vi "Init Actor Core.vi"(8 "error in (no error)":errorcluster, 11 "Measure Object in":refnum<class "Instrument Actor.lvclass">) -> (0 "error out":errorcluster, 3 "Measure Object out":refnum<class "Instrument Actor.lvclass">)   [LabVIEW 2021, in "Instrument Actor.lvclass"]
uses:
  Instrument Actor.lvclass
  Instrument Actor.lvclass/Instrument Actor.ctl
  Worker/Worker.lvclass
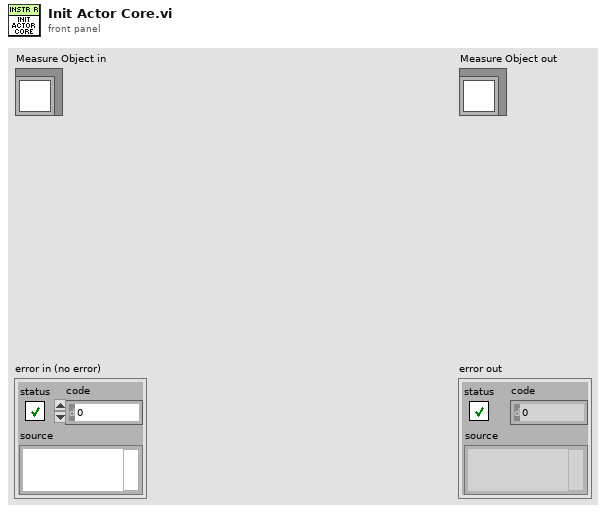
[diagram p1: front panel]
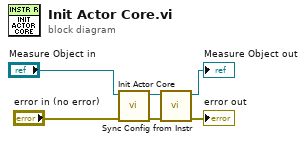
[diagram p0: block diagram]
diagram:
  n1 = call-parent "Init Actor Core.vi"("error in (no error)"="error in (no error)", "Measure Object in"="Measure Object in") -> ("error out"=w3:errorcluster, "Measure Object out"=w4:refnum<class "Instrument Actor.lvclass">)  [unwired: 8 in]
  n2 = call-dynamic "Sync Config from Instr.vi"("error in (no error)"=w3, "Instrument Actor in"=w4) -> ("error out"=→"error out":errorcluster, "Instrument Actor out"=→"Measure Object out":refnum<class "Instrument Actor.lvclass">)  [unwired: 8 in]
